vi "xxxx.vi"   [LabVIEW 2014]
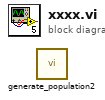
[diagram p0: block diagram]
diagram:
  n1 = call "generate_population2.vi"() -> ()  [unwired: 11 in, 1 out]
